vi "construct.vi"(8 "error in (no error)":errorcluster, 9 "configuration name":string, 10 "load config file?":bool=TRUE, 11 "GenericPlugin in":refnum<class "TrajectoryRK110916Throughput.lvclass">) -> (0 "error out":errorcluster, 3 "GenericPlugin out":refnum<class "TrajectoryRK110916Throughput.lvclass">)   [LabVIEW 2010, in "TrajectoryRK110916Throughput.lvclass"]
uses:
  TrajectoryRK110916Throughput.lvclass
  TrajectoryMG100122GenericFPGA/TrajectoryMG100122GenericFPGA/TrajectoryMG100122GenericFPGA.lvclass
  FPGAWrapper/GenericFPGAWrapper/GenericFPGAWrapper/GenericFPGAWrapper.lvclass
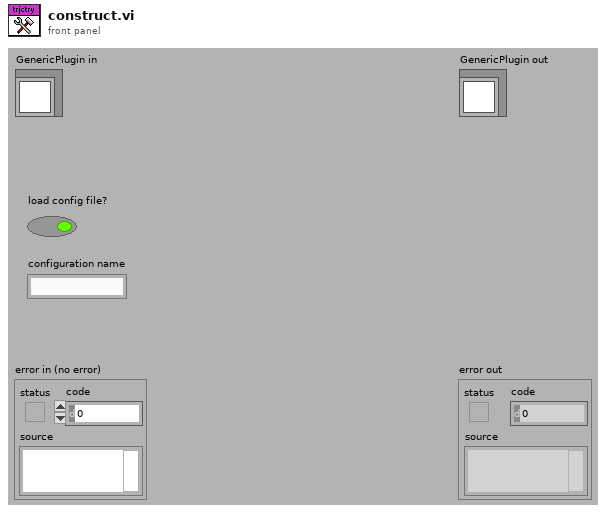
[diagram p1: front panel]
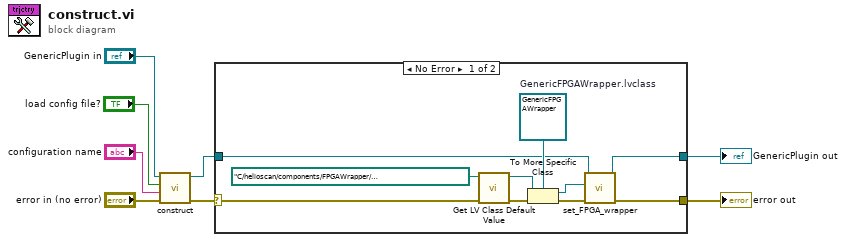
[diagram p0: block diagram]
diagram:
  n1 = call-parent "construct.vi"("error in (no error)"="error in (no error)", "configuration name"="configuration name", "load config file?"="load config file?", "GenericPlugin in"="GenericPlugin in") -> ("error out"=w4:errorcluster, "GenericPlugin out"=w3:refnum<class "TrajectoryRK110916Throughput.lvclass">)  [unwired: 6 in]
  n2 = case shown="No Error" w4 {
    selector: w4 -> [w18 w20]
    tunnel: w3 -> [w11 w19]
    tunnel: [w10 w19] -> w1
    tunnel: [w9 w20] -> w2
    frame No Error {
      w14 = refnum<class "GenericFPGAWrapper.lvclass"> refnum  # GenericFPGAWrapper.lvclass
      n3 = call <vilib>:"Get LV Class Default Value.vi"("error in (no error)"=w18, "class path"=path "C:/helioscan/components/FPGAWrapper/FPGAWrapperRK110909Throughput/FPGAWrapperRK110909Throughput/FPGAWrapperRK110909Throughput.lvclass") -> ("error out"=w16:errorcluster, "object"=w15:refnum<class>)  [unwired: 8 in]
      n4 = To More Specific Class(target class=w14, reference=w15, error in=w16) -> (specific class reference=w12:refnum<class "GenericFPGAWrapper.lvclass">, error out=w13:errorcluster)
      n5 = call-dynamic "set_FPGA_wrapper.vi"("error in (no error)"=w13, "GenericFPGAWrapper.lvclass"=w12, "TrajectoryMG100122GenericFPGA in"=w11) -> ("error out"=w9:errorcluster, "TrajectoryMG100122GenericFPGA out"=w10:refnum<class "TrajectoryRK110916Throughput.lvclass">)  [unwired: 7 in]
    }
    frame Error {
    }
  }
  "error out" <- w2
  "GenericPlugin out" <- w1
